vi "GripperAngle.vi"() -> ()   [LabVIEW 2017]
uses:
  global variable.vi
panel:
  out "x-y":i32
  in  "정지":bool
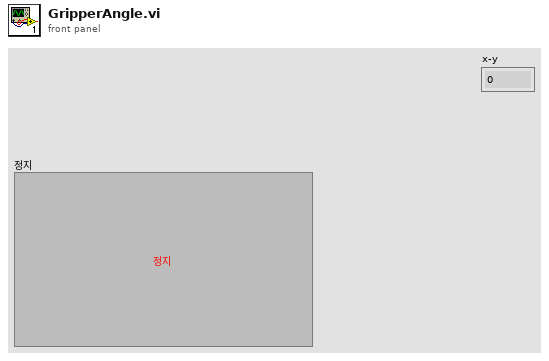
[diagram p1: front panel]
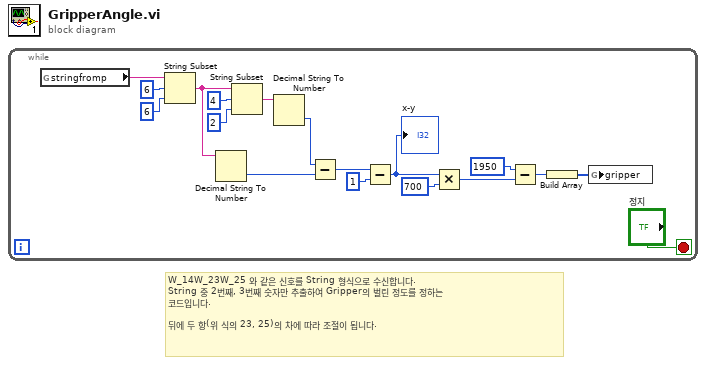
[diagram p0: block diagram]
diagram:
  # "W_14W_23W_25 와 같은 신호를 String 형식으로 수신합니다.\nString 중 2번째, 3번째 숫자만 추출하여 Gripper의 벌린 정도를 정하는\n코드입니다.\n\n뒤에 두 항(위 식의 23, 25)의 차에 따라 조절이 됩니다."
  n1 = while {
    stop <- "정지" stop-if-true
    n2 = global read "global variable.vi" "stringfromp"() -> (w11:string)
    n3 = String Subset(string=w11, offset (0)=6 ("오프셋(0)"), length (rest)=6 ("길이(나머지)")) -> (substring=w13:string)
    n4 = Decimal String To Number(string=w13) -> (number=w9:i32)  [unwired: 2 in, 1 out]
    n5 = String Subset(string=w13, offset (0)=4 ("오프셋(0)"), length (rest)=2 ("길이(나머지)")) -> (substring=w12:string)
    n6 = Decimal String To Number(string=w12) -> (number=w10:i32)  [unwired: 2 in, 1 out]
    n7 = Subtract(x=w10, y=w9) -> (x-y=w8:i32)
    n8 = Subtract(x=w8, y=1) -> (x-y=w5:i32)
    "x-y" <- w5
    n9 = Multiply(x=w5, y=700) -> (x*y=w2:i32)
    n10 = Subtract(x=1950, y=w2) -> (x-y=w1:i32)
    n11 = Build Array(w1) -> (w6:i32[])
    n12 = global write "global variable.vi" "gripper"(w6) -> ()
  }
